vi "Sleep.vi"(8 "error in (no error)":errorcluster, 11 "CIFCorePlugin in":refnum<class "CIFCorePlugin.lvclass">) -> (0 "error out":errorcluster, 3 "CIFCorePlugin out":refnum<class "CIFCorePlugin.lvclass">)   [LabVIEW 2021, in "CIFCorePlugin.lvclass"]
uses:
  CIFCorePlugin.lvclass
  CIFCorePlugin.lvclass/CIFCorePlugin.ctl
  CIFUtilities/CIFClocks/Typedef/Errors.ctl
  Accessors/Timestamps/Write Target Wake TS.vi
  Accessors/Get Time.vi
  Accessors/Timestamps/Read Running TS.vi
  Accessors/Read Iterations.vi
  Accessors/Read Timing Override.vi
  Accessors/Read Common Config.vi
  CIFUtilities/CIFClocks/Core/Get Time.vi
  CIFUtilities/CIFClocks/Time Conversion/LabVIEW Time to UTC Time.vi
  CIFCoreCommon/CIFCoreCommon.lvlib
  CIFUtilities/CIFClocks/CIFClocks.lvlib
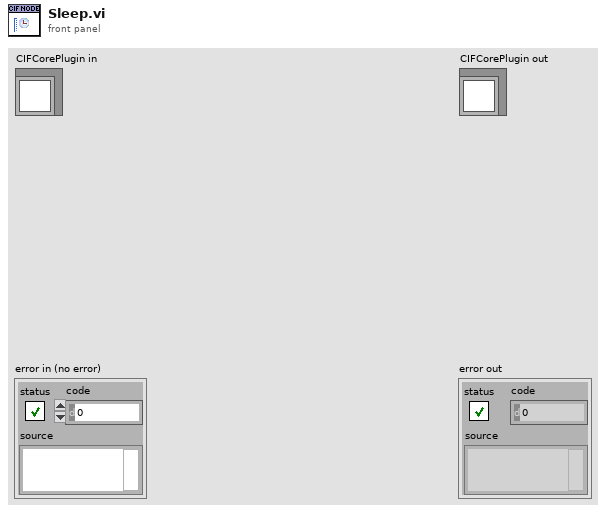
[diagram p1: front panel]
types:
  T1 = typedef "CIFCoreCommon.lvlib/Errors.ctl" = enum16{"Invalid Clock ID", "Long Sleep", "gRPC Server Not Found", "Config Parse", "Timestamp Wrap", "Delayed Execution"}
  T2 = typedef "CIFCoreCommon.lvlib/Timing Overrides.ctl" = cluster{"Override Timing":bool, "Skip Sleep":bool, "Period (s)":dbl}
  T3 = typedef "CIFCoreCommon.lvlib/Common Plugin Configuration.ctl" = cluster{"Period (s)":dbl, "Offset (us)":i32, "ClockID":u8, "Priority":i32, "Processor":i32}
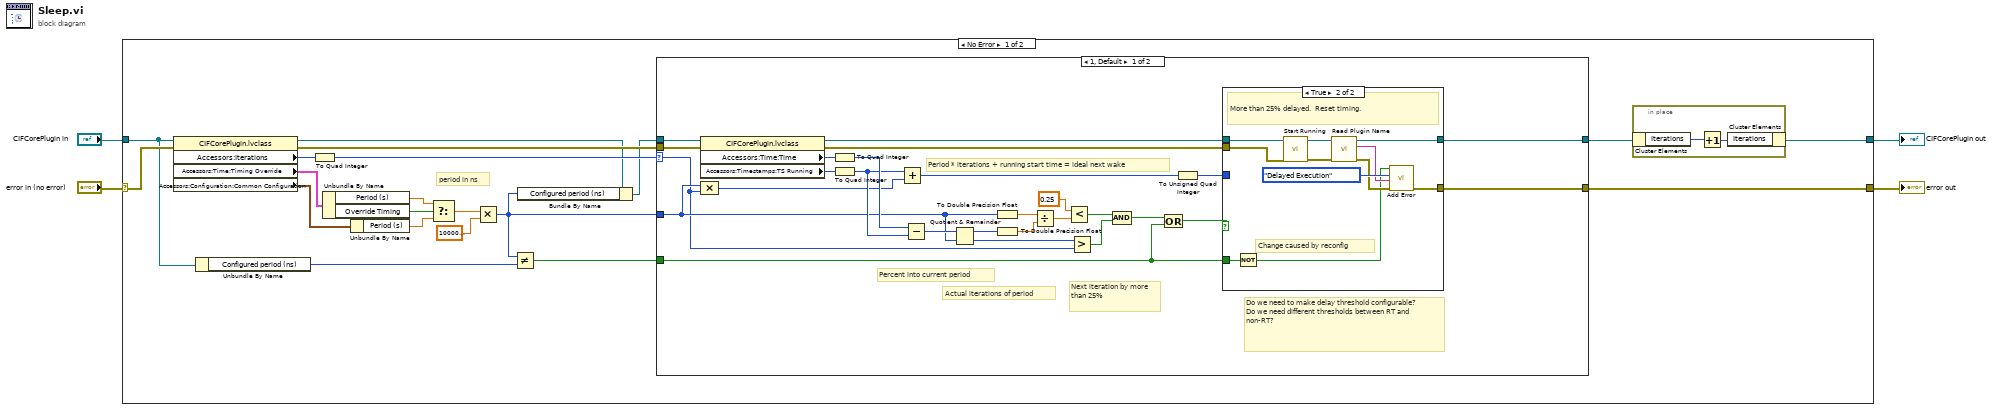
[diagram p0: block diagram]
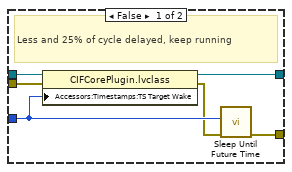
[diagram p2: hidden frame]
diagram:
  n1 = case shown="No Error" "error in (no error)" {
    selector: "error in (no error)" -> [w20 w74]
    tunnel: [w24 w74] -> w3
    tunnel: [w22 w73] -> w1
    tunnel: "CIFCorePlugin in" -> [w9 w73]
    frame No Error {
      # "period in ns"
      n2 = property class="CIFCorePlugin.lvclass"(reference=w9, error in=w20) -> (reference out=w7:refnum<class "CIFCorePlugin.lvclass">, error out=w21:errorcluster, "Accessors:Iterations"=w11:u32, "Accessors:Time:Timing Override"=w12:T2, "Accessors:Configuration:Common Configuration"=w15:T3)
      n3 = Unbundle By Name(w9) -> ("Configured period (ns)"=w8:i64)
      n4 = To Quad Integer(1:w11) -> (0:w10:i64)
      n5 = Unbundle By Name(w12) -> ("Period (s)"=w14:dbl, "Override Timing"=w16:bool)
      n6 = Unbundle By Name(w15) -> ("Period (s)"=w19:dbl)
      n7 = Select(t=w14, s=w16, f=w19) -> (s? t:f=w17:dbl)
      n8 = Multiply(x=w17, y=1000000000.0 ("x")) -> (x*y=w5:i64)
      n9 = Not Equal?(x=w5, y=w8) -> (x != y?=w13:bool)
      n10 = Bundle By Name(cluster=w7, "Configured period (ns)"=w5) -> (w6:refnum<class "CIFCorePlugin.lvclass">)
      n11 = case shown="1, Default" w10 {
        selector: w10 -> [w29 _]
        tunnel: [w40 w72] -> w23
        tunnel: w21 -> [w53 w71]
        tunnel: w6 -> [w52 w72]
        tunnel: [w39 w71] -> w24
        tunnel: w5 -> [w31 _]
        tunnel: w13 -> [w33 _]
        frame 1, Default {
          # "Percent into current period"
          # "Actual iterations of period"
          # "Next iteration by more than 25%"
          # "Do we need to make delay threshold configurable?  Do we need different thresholds between RT and non-RT?"
          # "Period * iterations + running start time = ideal next wake"
          n12 = property class="CIFCorePlugin.lvclass"(reference=w52, error in=w53) -> (reference out=w41:refnum<class "CIFCorePlugin.lvclass">, error out=w38:errorcluster, "Accessors:Time:Time"=w37:u64, "Accessors:Timestamps:TS Running"=w32:u64)
          n13 = Compound Arithmetic op=MULTIPLY(w31, w29) -> (w30:i64)
          n14 = To Quad Integer(1:w37) -> (0:w44:i64)
          n15 = To Quad Integer(1:w32) -> (0:w43:i64)
          n16 = Add(x=w43, y=w30) -> (x+y=w28:i64)
          n17 = Subtract(x=w44, y=w43) -> (x-y=w42:i64)
          n18 = Quotient & Remainder(x=w42, y=w31) -> (x-y*floor(x/y)=w51:i64, floor(x/y)=w36:i64)
          n19 = To Double Precision Float(number=w31) -> (double precision float=w49:dbl)
          n20 = To Double Precision Float(number=w51) -> (double precision float=w50:dbl)
          n21 = Divide(x=w49, y=w50) -> (x/y=w48:dbl)
          n22 = Less?(x=0.25 ("y"), y=w48) -> (x < y?=w46:bool)
          n23 = Greater?(x=w36, y=w29) -> (0:w45:bool)
          n24 = Compound Arithmetic op=AND(w46, w45) -> (w35:bool)
          n25 = Compound Arithmetic op=OR(w35, w33) -> (w34:bool)
          n26 = To Unsigned Quad Integer(1:w28) -> (0:w27:u64)
          n27 = case shown="True" w34 {
            tunnel: w41 -> [w58 w70]
            tunnel: [w54 w65] -> w40
            tunnel: w38 -> [w57 w69]
            tunnel: [w59 w64] -> w39
            tunnel: w33 -> [_ w61]
            tunnel: w27 -> [w56 _]
            frame False {
              # "Less and 25% of cycle delayed, keep running"
              n28 = property class="CIFCorePlugin.lvclass"(reference=w58, error in=w57, "Accessors:Timestamps:TS Target Wake"=w56) -> (reference out=w54:refnum<class "CIFCorePlugin.lvclass">, error out=w55:errorcluster)
              n29 = call "Sleep Until Future Time.vi"("error in (no error)"=w55, "Wake Time"=w56) -> ("error out"=w59:errorcluster)  [unwired: 9 in]
            }
            frame True {
              # "Change caused by reconfig"
              # "More than 25% delayed.  Reset timing."
              n30 = Not(x=w61) -> (.not. x?=w60:bool)
              n31 = call "Start Running.vi"("error in (no error)"=w69, "CIFCorePlugin in"=w70) -> ("error out"=w62:errorcluster, "CIFCorePlugin out"=w63:refnum<class "CIFCorePlugin.lvclass">)  [unwired: 8 in]
              n32 = call "Read Plugin Name.vi"("error in (no error)"=w62, "CIFTemplateNode in"=w63) -> ("error out"=w66:errorcluster, "Plugin Name"=w67:string, "CIFTemplateNode out"=w65:refnum<class "CIFCorePlugin.lvclass">)  [unwired: 7 in]
              n33 = call "Add Error.vi"("error in (no error)"=w66, "String to Append"=w67, "Error"=Errors."Delayed Execution", "Insert Error"=w60) -> ("error out"=w64:errorcluster)  [unwired: 7 in]
            }
          }
        }
        frame 0 {
          # "First execution when entering running state.  Don't sleep"
        }
      }
      n34 = in-place {
        n35 = in-place-cluster #1(w23) -> ("Iterations"=w25:i64)
        n36 = Increment(x=w25) -> (x+1=w26:i64)
        n37 = in-place-cluster #1("Iterations"=w26) -> (w22:refnum<class "CIFCorePlugin.lvclass">)
      }
    }
    frame Error {
    }
  }
  "error out" <- w3
  "CIFCorePlugin out" <- w1
